vi "DuplicateFrame.vi"(7 "Replace FrameName if found? (T)":bool=TRUE, 8 "error in (no error)":errorcluster, 9 "New FrameName":string, 10 "FrameName to duplicate":string, 11 "CaseStructure Ref":refnum<vi>) -> (0 "error out":errorcluster, 1 "New Frame":refnum<vi>, 3 "CaseStructure Ref":refnum<vi>)   [LabVIEW 2019, in "BlueUtilityScripts.lvlib"]
uses:
  BlueUtilityScripts.lvlib
  <vilib>/Utility/error.llb/Error Cluster From Error Code.vi
  <vilib>/ErrorRing/Error Ring.xnode
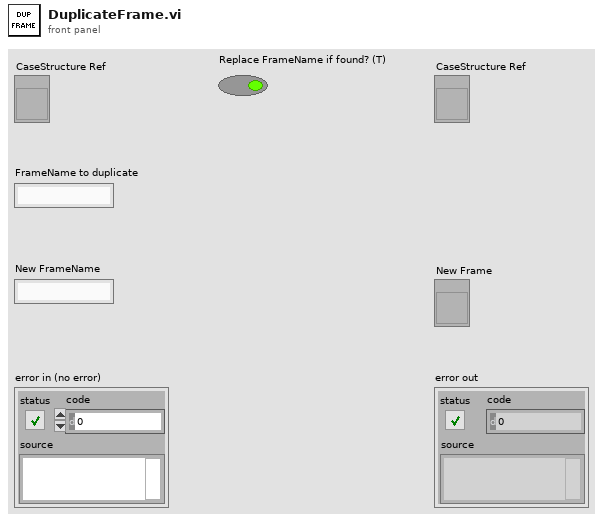
[diagram p1: front panel]
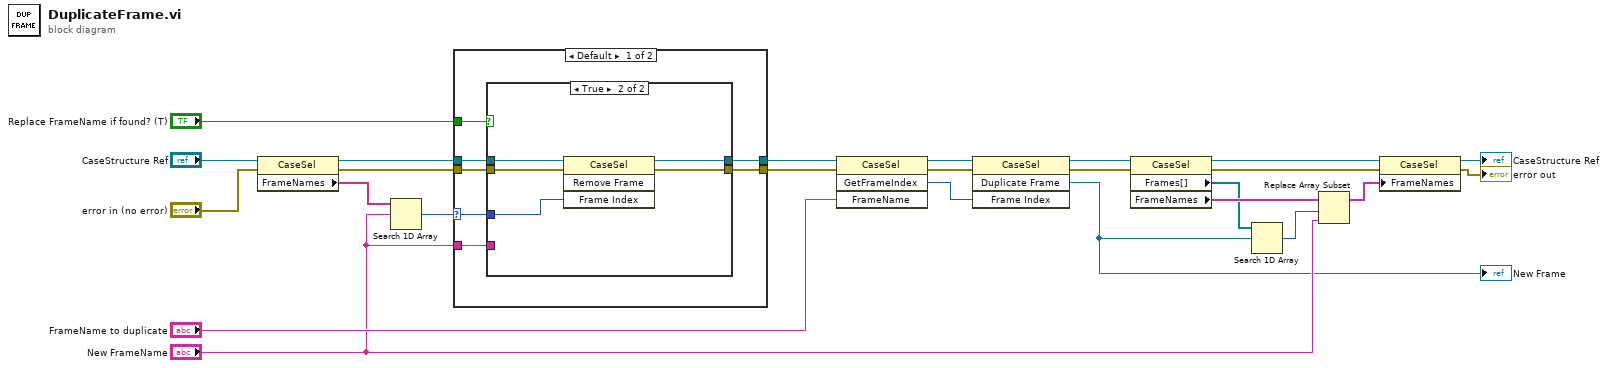
[diagram p0: block diagram]
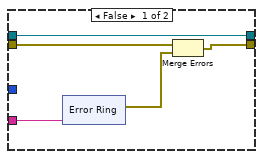
[diagram p2: hidden frame]
diagram:
  n1 = property class="CaseSel"(reference="CaseStructure Ref", error in="error in (no error)") -> (reference out=w22:refnum<vi>, error out=w20:errorcluster, "FrameNames"=w24:string[])
  n2 = Search 1D Array(1D array=w24, element="New FrameName") -> (index of element=w23:i32)  [unwired: 1 in]
  n3 = case shown="Default" w23 {
    selector: w23 -> [w30 _]
    tunnel: w22 -> [w31 w51]
    tunnel: "Replace FrameName if found? (T)" -> [w32 _]
    tunnel: w20 -> [w29 w50]
    tunnel: "New FrameName" -> [w28 _]
    tunnel: [w27 w51] -> w18
    tunnel: [w26 w50] -> w16
    frame Default {
      n4 = case shown="True" w32 {
        tunnel: w31 -> [w33 w49]
        tunnel: w30 -> [_ w48]
        tunnel: w29 -> [w36 w47]
        tunnel: w28 -> [w37 _]
        tunnel: [w34 w46] -> w26
        tunnel: [w33 w45] -> w27
        frame False {
          n5 = xnode "Error Ring"("parameter 0"=w37) -> ("error out"=w35:errorcluster)
          n6 = Merge Errors(w36, w35) -> (w34:errorcluster)
        }
        frame True {
          n7 = invoke class="CaseSel" method="Remove Frame"(reference=w49, error in=w47, "Frame Index"=w48) -> (reference out=w45:refnum<vi>, error out=w46:errorcluster)  [unwired: 1 in, 2 out]
        }
      }
    }
    frame -1 {
    }
  }
  n8 = invoke class="CaseSel" method="GetFrameIndex"(reference=w18, error in=w16, "FrameName"="FrameName to duplicate") -> (reference out=w15:refnum<vi>, error out=w13:errorcluster, "GetFrameIndex"=w14:i32)  [unwired: 1 in, 1 out]
  n9 = invoke class="CaseSel" method="Duplicate Frame"(reference=w15, error in=w13, "Frame Index"=w14) -> (reference out=w12:refnum<vi>, error out=w11:errorcluster, "Duplicate Frame"=w4:refnum<vi>)  [unwired: 1 in, 1 out]
  "New Frame" <- w4
  n10 = property class="CaseSel"(reference=w12, error in=w11) -> (reference out=w7:refnum<vi>, error out=w6:errorcluster, "Frames[]"=w2:refnum<vi>[], "FrameNames"=w10:string[])
  n11 = Search 1D Array(1D array=w2, element=w4) -> (index of element=w9:i32)  [unwired: 1 in]
  n12 = Replace Array Subset(array=w10, new element="New FrameName", index=w9) -> (w5:string[])
  n13 = property class="CaseSel"(reference=w7, error in=w6, "FrameNames"=w5) -> (reference out=→"CaseStructure Ref":refnum<vi>, error out=→"error out":errorcluster)
